vi "LowerCuffButton.vi"(0 "error in":errorcluster, 2 "Side":T1, 3 "node":string) -> (1 "error out":errorcluster, 4 "Digital IO State":cluster{"state":i8, "is input only":bool})   [LabVIEW 2013]
uses:
  ROS/Code/SubVIs/BaxterSide.ctl
panel:
  out "Reply":string
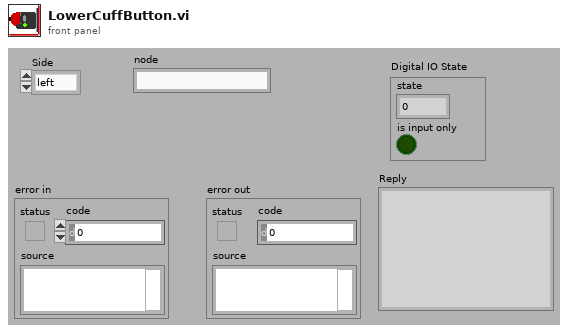
[diagram p1: front panel]
types:
  T1 = typedef "BaxterSide.ctl" = enum16{"left", "right"}
  T2 = typedef "_ROSControl.ctl" = cluster{"topic port":u16, "Node":string, "topic":string, "type":string, "node port":u32, "error ":errorcluster, "Direction":T3, "APIs":string[]}
  T3 = typedef "_ROSDirection.ctl" = enum16{"Node", "Publisher", "Subscriber", "Service Client"}
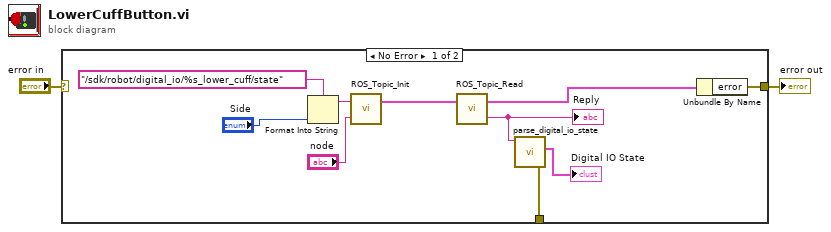
[diagram p0: block diagram]
diagram:
  n1 = case shown="No Error" "error in" {
    selector: "error in" -> [_ w13]
    tunnel: [w12 w13] -> w2
    tunnel: [w4 _] -> _
    frame No Error {
      n2 = Format Into String(format string="/sdk/robot/digital_io/%s_lower_cuff/state" ("topic"), "Side") -> (resulting string=w7:string)  [unwired: 2 in, 1 out]
      n3 = call "ROS_Topic_Init.vi"("node"="node", "topic"=w7) -> ("ROS out"=w10:T2)  [unwired: 1 in]
      n4 = call "ROS_Topic_Read.vi"("ROS in"=w10) -> ("Reply"=w6:string, "ROS out"=w9:T2)  [unwired: 1 in]
      "Reply" <- w6
      n5 = call "parse_digital_io_state.vi"("msg in"=w6) -> ("error out"=w4:errorcluster, "Digital IO State"=→"Digital IO State":cluster{"state":i8, "is input only":bool})  [unwired: 4 in, 1 out]
      n6 = Unbundle By Name(w9) -> ("error"=w12:errorcluster)
    }
    frame Error {
    }
  }
  "error out" <- w2
